vi "Entry.vi"(8 "error in (no error)":errorcluster, 11 "New State":refnum<class "Running Command.lvclass">) -> (0 "error out":errorcluster, 3 "State out":refnum<class "Running Command.lvclass">)   [LabVIEW 2014, in "Robot Actor Framework.lvlib" / "Command Processor Actor.lvlib" / "Running Command.lvclass"]
doc: "This is an abstract method. Override this method to define the behavior when you enter the state."
uses:
  Running Command.lvclass
  Command Processor Actor Class/Command Processor States.ctl
  <vilib>/ActorFramework/Message Enqueuer/Message Priority.ctl
  <vilib>/ActorFramework/Actor/Actor.lvclass/Actor.ctl
  <vilib>/ActorFramework/Message Enqueuer/Message Enqueuer.lvclass/Message Enqueuer.ctl
  <vilib>/ActorFramework/Message Enqueuer/Init from Existing Queue.vi
  <vilib>/ActorFramework/Message Enqueuer/Enqueue.vi
  <vilib>/ActorFramework/Message Priority Queue/Priority Enqueue.vi
  <vilib>/ActorFramework/Message Enqueuer/Message Enqueuer.lvclass
  Command Processor Actor Messages/Go To Stopping Command Msg/Go To Stopping Command Msg.lvclass
  Command Processor Actor Class/Command Processor Actor.lvclass
  <vilib>/ActorFramework/Actor/Actor.lvclass
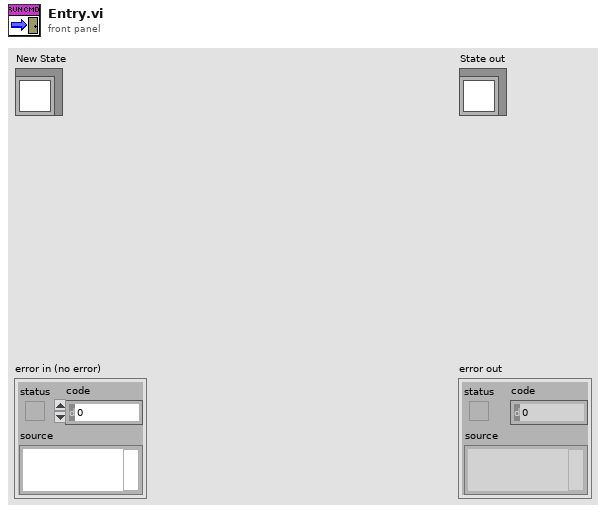
[diagram p1: front panel]
types:
  T1 = typedef "Robot Actor Framework.lvlib/Command Processor Actor.lvlib/Command Processor Actor.lvclass/Command Processor States.ctl" = enum16{"Unknown", "No Command", "Running Command", "Starting Command", "Stopping Command", "Finishing Command"}
  T2 = typedef "Actor Framework.lvlib/Message Enqueuer.lvclass/Message Priority.ctl" = enum16{"Low", "Normal", "High"}
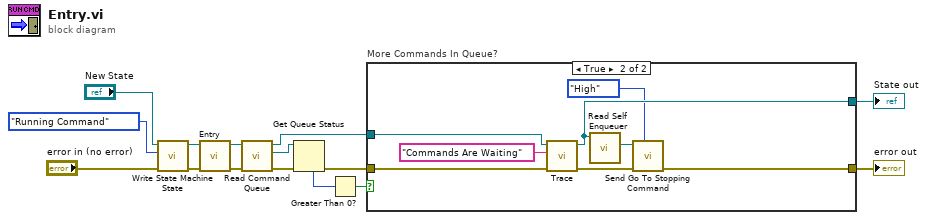
[diagram p0: block diagram]
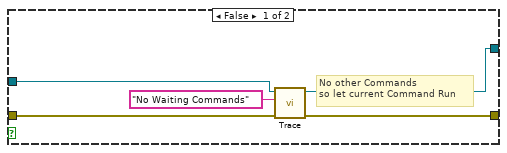
[diagram p2: hidden frame]
diagram:
  n1 = call-dynamic "Write State Machine State.vi"("error in (no error)"="error in (no error)", "Command Processor State"=Command_Processor_States."Running Command", "Command Processor Actor in"="New State") -> ("error out"=w4:errorcluster, "Command Processor Actor out"=w2:refnum<class "Running Command.lvclass">)  [unwired: 7 in]
  n2 = call-parent "Entry.vi"("error in (no error)"=w4, "New State"=w2) -> ("error out"=w9:errorcluster, "State out"=w11:refnum<class "Running Command.lvclass">)  [unwired: 8 in]
  n3 = call-dynamic "Read Command Queue.vi"("error in (no error)"=w9, "Command Processor Actor in"=w11) -> ("error out"=w8:errorcluster, "Queued Commands"=w15:refnum<queue>, "Command Processor Actor out"=w12:refnum<class "Running Command.lvclass">)  [unwired: 7 in]
  n4 = Get Queue Status(queue=w15, error in (no error)=w8) -> (error out=w7:errorcluster, # elements in queue=w14:i32)  [unwired: 1 in, 6 out]
  n5 = Greater Than 0?(x=w14) -> (x > 0?=w13:bool)
  n6 = case "More Commands In Queue?" shown="True" w13 {
    tunnel: w12 -> [w20 w28]
    tunnel: [w19 w25] -> w10
    tunnel: w7 -> [w17 w27]
    tunnel: [w16 w22] -> w6
    frame False {
      # "No other Commands\nso let current Command Run"
      n7 = call-dynamic "Trace.vi"("error in (no error)"=w17, "Command Processor Action"="No Waiting Commands", "Command Processor Actor in"=w20) -> ("error out"=w16:errorcluster, "Command Processor Actor out"=w19:refnum<class "Running Command.lvclass">)  [unwired: 7 in]
    }
    frame True {
      n8 = call-dynamic "Trace.vi"("error in (no error)"=w27, "Command Processor Action"="Commands Are Waiting", "Command Processor Actor in"=w28) -> ("error out"=w23:errorcluster, "Command Processor Actor out"=w25:refnum<class "Running Command.lvclass">)  [unwired: 7 in]
      n9 = call <vilib>:"Read Self Enqueuer.vi"("Actor"=w25) -> ("Self Enqueuer"=w24:refnum<class "Message Enqueuer.lvclass">)  [unwired: 10 in]
      n10 = call "Send Go To Stopping Command.vi"("Message Priority (Normal)"=Message_Priority."High", "error in (no error)"=w23, "Message Enqueuer"=w24) -> ("error out"=w22:errorcluster)  [unwired: 7 in, 1 out]
    }
  }
  "error out" <- w6
  "State out" <- w10
